vi "matlab_TI2_filterArraySet.vi"(8 "error in":errorcluster, 10 "Filter index":i32, 11 "Filter array":dbl[](array[numeric])) -> (0 "error out":errorcluster, 2 "Current filter":dbl)   [LabVIEW 2018]
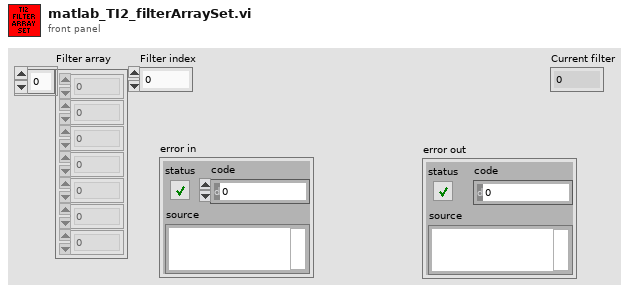
[diagram p1: front panel]
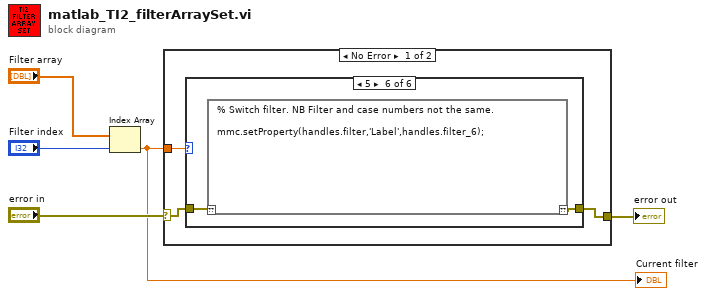
[diagram p0: block diagram]
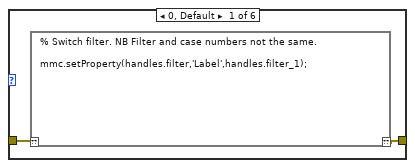
[diagram p2: hidden frame]
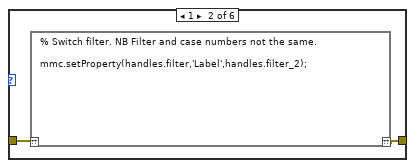
[diagram p3: hidden frame]
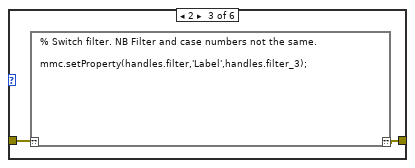
[diagram p4: hidden frame]
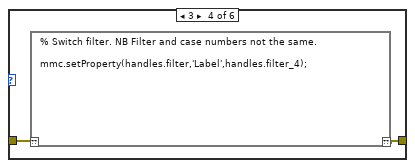
[diagram p5: hidden frame]
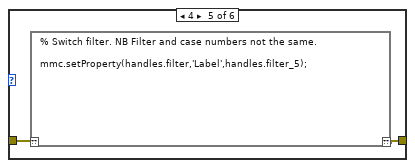
[diagram p6: hidden frame]
diagram:
  n1 = Index Array(array="Filter array", index="Filter index") -> (element=w1:dbl)
  "Current filter" <- w1
  n2 = case shown="No Error" "error in" {
    selector: "error in" -> [w7 w21]
    tunnel: [w6 w21] -> w4
    tunnel: w1 -> [w8 _]
    frame No Error {
      n3 = case shown="5" w8 {
        tunnel: w7 -> [w10 w12 w14 w16 w18 w20]
        tunnel: [w9 w11 w13 w15 w17 w19] -> w6
        frame 0, Default {
          n4 = script code="% Switch filter. NB Filter and case numbers not the same.\n\nmmc.setProperty(handles.filter,'Label',handles.filter_1);"("??"=w10) -> ("??"=w9:errorcluster)
        }
        frame 1 {
          n5 = script code="% Switch filter. NB Filter and case numbers not the same.\n\nmmc.setProperty(handles.filter,'Label',handles.filter_2);"("??"=w12) -> ("??"=w11:errorcluster)
        }
        frame 2 {
          n6 = script code="% Switch filter. NB Filter and case numbers not the same.\n\nmmc.setProperty(handles.filter,'Label',handles.filter_3);"("??"=w14) -> ("??"=w13:errorcluster)
        }
        frame 3 {
          n7 = script code="% Switch filter. NB Filter and case numbers not the same.\n\nmmc.setProperty(handles.filter,'Label',handles.filter_4);"("??"=w16) -> ("??"=w15:errorcluster)
        }
        frame 4 {
          n8 = script code="% Switch filter. NB Filter and case numbers not the same.\n\nmmc.setProperty(handles.filter,'Label',handles.filter_5);"("??"=w18) -> ("??"=w17:errorcluster)
        }
        frame 5 {
          n9 = script code="% Switch filter. NB Filter and case numbers not the same.\n\nmmc.setProperty(handles.filter,'Label',handles.filter_6);"("??"=w20) -> ("??"=w19:errorcluster)
        }
      }
    }
    frame Error {
    }
  }
  "error out" <- w4
